vi "Pass Recovery State Machine.vi"   [LabVIEW 2013]
uses:
  typedefs/State Machine/subStates.ctl
  typedefs/fg_typedef.ctl
  typedefs/DevRef Type.ctl
panel:
  # "A State Machine to Handle Recovering From a Failed Pass"
types:
  T1 = typedef "subStates.ctl" = enum16{"null", "wait", "driver control", "auto", "manual override", "hold position", "rotate", "pickup", "pass", "recover pass", "load", "goto shoot", "shoot high goal", "shoot low goal", "cancel arm", "cancel shooter", "end", "test"}
  T2 = typedef "DevRef Type.ctl" = enum16{"Shooter Solenoid", "Latch Solenoid", "Right Up Sensor", "Right Down Sensor", "Hold Sensor", "2 Ball Switch", "Arm Encoder"}
  T3 = typedef "fg_typedef.ctl" = enum16{"Get", "Set"}
  T4 = typedef "WPI_EncoderDevRef.ctl" = cluster{"DevStatus":errorcluster, "EncoderIndex":T5, "CounterIndex":T6, "DistancePerCount":dbl, "Decoding Type":T7}
  T5 = typedef "FPGA_EncoderIdx.ctl" = enum8{"Enc 0", "Enc 1", "Enc 2", "Enc 3", "Invalid"}
  T6 = typedef "FPGA_CounterCtrSystemIndex.ctl" = enum8{"Ctr 0", "Ctr 1", "Ctr 2", "Ctr 3", "Ctr 4", "Ctr 5", "Ctr 6", "Ctr 7", "Invalid"}
  T7 = typedef "WPI_EncoderType.ctl" = enum16{"1x", "2x", "4x"}
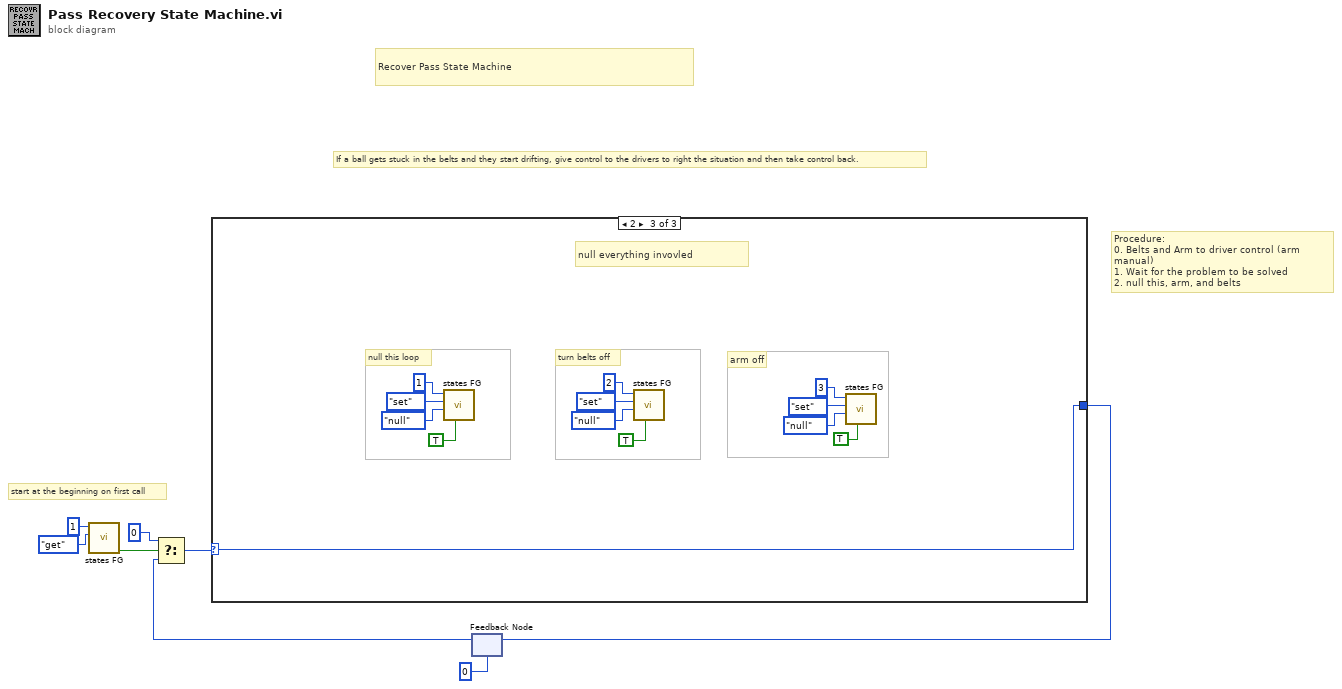
[diagram p0: block diagram]
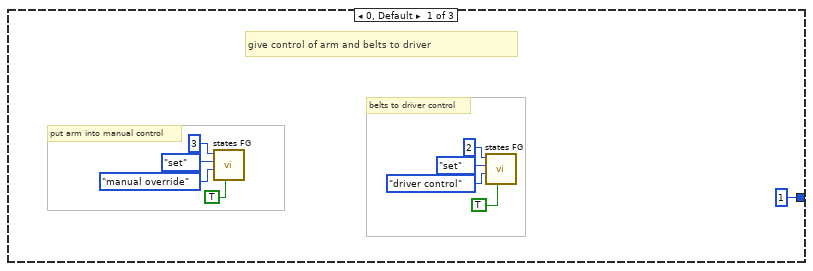
[diagram p2: hidden frame]
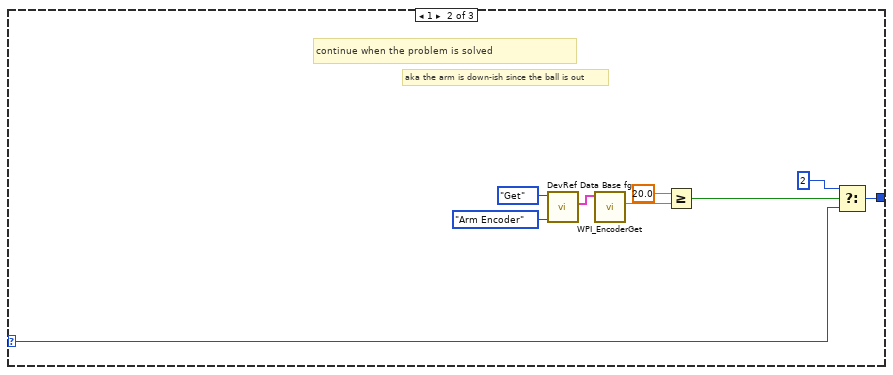
[diagram p3: hidden frame]
diagram:
  # "If a ball gets stuck in the belts and they start drifting, give control to the drivers to right the situation and then take control back."
  # "Procedure:\n0. Belts and Arm to driver control (arm manual)\n1. Wait for the problem to be solved\n2. null this, arm, and belts"
  # "Recover Pass State Machine"
  # "start at the beginning on first call"
  n1 = call "states FG.vi"("menu (get)"=enum16{"set", "get"}."get", "Loop ID"=1) -> ("first call?"=w1:bool)  [unwired: 6 in, 3 out]
  n2 = feedback #1(u8 0) -> (w4:u8)
  n3 = Select(t=u8 0, s=w1, f=w4) -> (s? t:f=w3:u8)
  n4 = case shown="2" w3 {
    selector: w3 -> [_ w26 w27]
    tunnel: [u8 1 ("t") w25 w27] -> w7
    frame 0, Default {
      # "put arm into manual control"
      # "belts to driver control"
      # "give control of arm and belts to driver"
      n5 = call "states FG.vi"("exit in"=TRUE, "subState in"=subStates."manual override", "menu (get)"=enum16{"set", "get"}."set", "Loop ID"=3) -> ()  [unwired: 4 in, 4 out]
      n6 = call "states FG.vi"("exit in"=TRUE, "subState in"=subStates."driver control", "menu (get)"=enum16{"set", "get"}."set", "Loop ID"=2) -> ()  [unwired: 4 in, 4 out]
    }
    frame 1 {
      # "aka the arm is down-ish since the ball is out"
      # "continue when the problem is solved"
      n7 = call "DevRef Data Base fg.vi"("DevRef to Get"=DevRef_Type."Arm Encoder", "Menu"=fg_typedef."Get") -> ("Selected Encoder"=w21:T4)  [unwired: 2 in, 5 out]
      n8 = call <vilib>:"WPI_EncoderGet.vi"("EncoderDevRef"=w21) -> ("Distance"=w20:dbl)  [unwired: 5 in, 5 out]
      n9 = Greater Or Equal?(x=20.0, y=w20) -> (x >= y?=w18:bool)
      n10 = Select(t=u8 2, s=w18, f=w26) -> (s? t:f=w25:u8)
    }
    frame 2 {
      # "turn belts off"
      # "arm off"
      # "null this loop"
      # "null everything invovled"
      n11 = call "states FG.vi"("exit in"=TRUE, "subState in"=subStates."null", "menu (get)"=enum16{"set", "get"}."set", "Loop ID"=1) -> ()  [unwired: 4 in, 4 out]
      n12 = call "states FG.vi"("exit in"=TRUE, "subState in"=subStates."null", "menu (get)"=enum16{"set", "get"}."set", "Loop ID"=2) -> ()  [unwired: 4 in, 4 out]
      n13 = call "states FG.vi"("exit in"=TRUE, "subState in"=subStates."null", "menu (get)"=enum16{"set", "get"}."set", "Loop ID"=3) -> ()  [unwired: 4 in, 4 out]
    }
  }
  n14 = feedback-in #1(w7) -> ()
